vi "ConfigParams - Set - TCP.vi"(8 "error in (no error)":errorcluster, 9 "TCPLoopTime_mS":u32=10, 10 "TCPCommandPort":u16=12345, 11 "Ethernet in":refnum<class "ENET_BS1201.lvclass">) -> (0 "error out":errorcluster, 3 "Ethernet out":refnum<class "ENET_BS1201.lvclass">)   [LabVIEW 2021, in "BS120x Driver.lvlib" / "ENET_BS1201.lvclass"]
uses:
  ENET_BS1201.lvclass
panel:
  # "[TCP]\nTCPCommandPort = 12345\nTCPTimeout_ms = 2000\nTCPLoopTime_ms = 10"
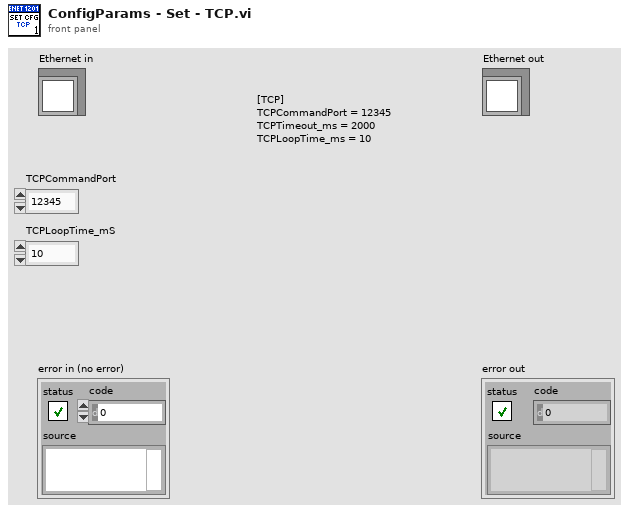
[diagram p1: front panel]
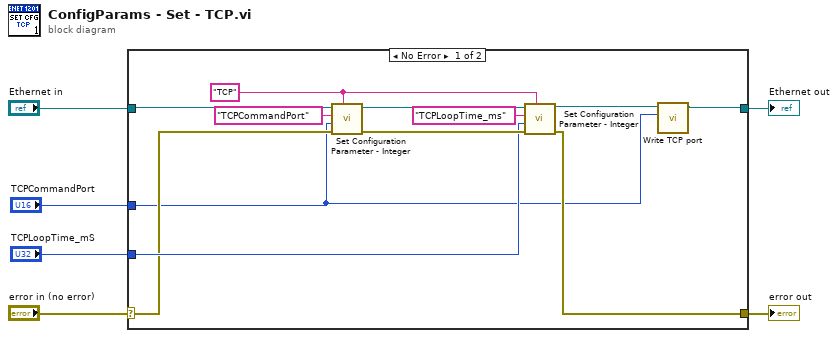
[diagram p0: block diagram]
diagram:
  n1 = case shown="No Error" "error in (no error)" {
    selector: "error in (no error)" -> [w10 w20]
    tunnel: [w12 w20] -> w5
    tunnel: [w7 w19] -> w3
    tunnel: "Ethernet in" -> [w11 w19]
    tunnel: "TCPCommandPort" -> [w8 _]
    tunnel: "TCPLoopTime_mS" -> [w13 _]
    frame No Error {
      w15 = "TCP" ("Section")
      n2 = call-dynamic "Set Configuration Parameter - Integer.vi"("Section"=w15, "error in (no error)"=w10, "Value"=w8, "Key"="TCPCommandPort", "Ethernet in"=w11) -> ("error out"=w16:errorcluster, "Ethernet out"=w17:refnum<class "ENET_BS1201.lvclass">)  [unwired: 5 in]
      n3 = call-dynamic "Set Configuration Parameter - Integer.vi"("Section"=w15, "error in (no error)"=w16, "Value"=w13, "Key"="TCPLoopTime_ms", "Ethernet in"=w17) -> ("error out"=w12:errorcluster, "Ethernet out"=w9:refnum<class "ENET_BS1201.lvclass">)  [unwired: 5 in]
      n4 = call-dynamic "Write TCP port.vi"("TCP port"=w8, "ENET_BS120x in"=w9) -> ("ENET_BS120x out"=w7:refnum<class "ENET_BS1201.lvclass">)  [unwired: 8 in, 1 out]
    }
    frame Error {
    }
  }
  "error out" <- w5
  "Ethernet out" <- w3
